vi "Ignore Comment.vi"(8 "Error In":errorcluster, 11 "Parser In":refnum<class "Lexer.lvclass">) -> (0 "Error Out":errorcluster, 3 "Parser Out":refnum<class "Lexer.lvclass">)   [LabVIEW 2018, in "Toolkit.lvlib" / "Lexer.lvclass"]
uses:
  Lexer.lvclass
  Lexer.lvclass/Lexer.ctl
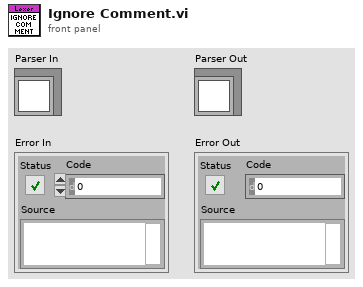
[diagram p1: front panel]
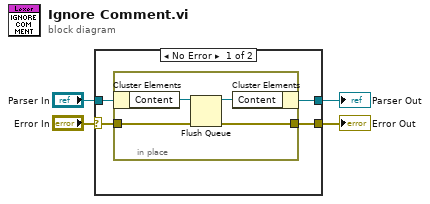
[diagram p0: block diagram]
diagram:
  n1 = case shown="No Error" "Error In" {
    selector: "Error In" -> [w5 w13]
    tunnel: [w8 w13] -> w4
    tunnel: [w7 w14] -> w3
    tunnel: "Parser In" -> [w6 w14]
    frame No Error {
      n2 = in-place {
        in-place-border: [w10] -> w8
        in-place-border: w5 -> [w9]
        n3 = in-place-cluster #1(w6) -> ("Content"=w12:refnum<queue>)
        n4 = Flush Queue(queue=w12, error in (no error)=w9) -> (queue out=w11:refnum<queue>, error out=w10:errorcluster)  [unwired: 1 out]
        n5 = in-place-cluster #1("Content"=w11) -> (w7:refnum<class "Lexer.lvclass">)
      }
    }
    frame Error {
    }
  }
  "Error Out" <- w4
  "Parser Out" <- w3
